vi "ProdaNG.Product.Add.vi"(8 "error in (no error)":errorcluster, 10 "Product":T1, 11 "dbHandle":i32) -> (0 "error out":errorcluster, 2 "Product out":T1, 3 "dbHandle":i32)   [LabVIEW 2016]
doc: "This function creates a new Product out of a prefilled product structure.\nParameter:\nhandle is an Integer, which is returned by the function Login() at the creation of a new connection.\nproduct is a pointer on a product structure, which elements must be prefilled. The structure must be defined and filled in the calling program. Nearly all elements of the structure must be set to reasonable values. The element id is filled by the DLL with a new Id for the created record, if the returncode is 0. The element crTime is being filled by the DLL automatically. The elements mdTime and mdProcessStepId are not being filled.\nThe function checks if a product with the passed WabcoPartId and serial number already exists and returns this. In this case no new product record is created.\nReturncodes:\n0 No error\n234 (ERROR_MORE_DATA) in case that the product already exists. This is no error and the product structure is returned with the existing product. \n< 0 ORACLE Error code\n6 (ERROR_INVALID_HANDLE) in case of an invalid handle"
uses:
  Controls/ProdaNG.Product.ctl
  Controls/ProdaNG.ProductSize.ctl
  prodllNG.dll
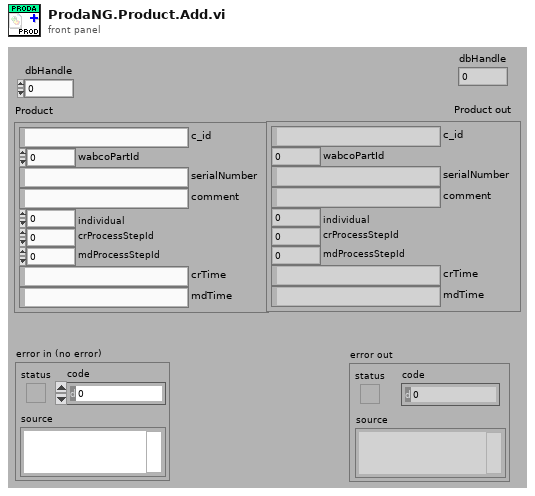
[diagram p1: front panel]
types:
  T1 = typedef "ProdaNG.Product.ctl" = cluster{"c_id":string, "wabcoPartId":i32, "serialNumber":string, "comment":string, "individual":i32, "crProcessStepId":i32, "mdProcessStepId":i32, "crTime":string, "mdTime":string}
  T2 = typedef "ProdaNG.ProductSize.ctl" = cluster{"c_id":i32, "wabcoPartId":i32, "serialNumber":i32, "comment":i32, "individual":i32, "crProcessStepId":i32, "mdProcessStepId":i32, "crTime":i32, "mdTime":i32}
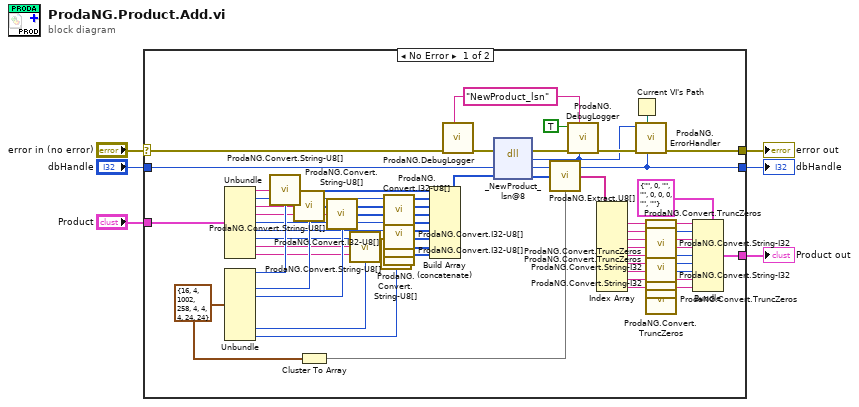
[diagram p0: block diagram]
diagram:
  n1 = case shown="No Error" "error in (no error)" {
    selector: "error in (no error)" -> [w60 w68]
    tunnel: [w66 w68] -> w5
    tunnel: "dbHandle" -> [w64 w67]
    tunnel: [w63 w67] -> w3
    tunnel: "Product" -> [w51 _]
    tunnel: [w30 _] -> w1
    frame No Error {
      w7 = T2 {"c_id"=16, "wabcoPartId"=4, "serialNumber"=1002, "comment"=258, "individual"=4, "crProcessStepId"=4, "mdProcessStepId"=4, "crTime"=24, "mdTime"=24} ("ProductSize")
      w61 = "NewProduct_lsn" ("cmd")
      n2 = Unbundle(w51) -> ("c_id"=w55:string, "wabcoPartId"=w26:i32, "serialNumber"=w25:string, "comment"=w24:string, "individual"=w18:i32, "crProcessStepId"=w16:i32, "mdProcessStepId"=w14:i32, "crTime"=w13:string, "mdTime"=w10:string)
      n3 = Unbundle(w7) -> ("c_id"=w53:i32, "serialNumber"=w23:i32, "comment"=w22:i32, "crTime"=w11:i32, "mdTime"=w9:i32)  [unwired: 4 out]
      n4 = call "ProdaNG.Convert.String-U8[].vi"("Input String"=w55, "Size"=w53) -> ("Output"=w52:u8[])
      n5 = call "ProdaNG.Convert.String-U8[].vi"("Input String"=w25, "Size"=w23) -> ("Output"=w20:u8[])
      n6 = Cluster To Array(cluster=w7) -> (array=w54:i32[])
      n7 = call "ProdaNG.Convert.String-U8[].vi"("Input String"=w24, "Size"=w22) -> ("Output"=w21:u8[])
      n8 = call "ProdaNG.Convert.String-U8[].vi"("Input String"=w13, "Size"=w11) -> ("Output"=w12:u8[])
      n9 = call "ProdaNG.Convert.String-U8[].vi"("Input String"=w10, "Size"=w9) -> ("Output"=w8:u8[])
      n10 = call "ProdaNG.Convert.I32-U8[].vi"("32bit integer"=w26) -> ("unsigned byte array"=w27:u8[])  [unwired: 10 in]
      n11 = call "ProdaNG.Convert.I32-U8[].vi"("32bit integer"=w18) -> ("unsigned byte array"=w19:u8[])  [unwired: 10 in]
      n12 = call "ProdaNG.Convert.I32-U8[].vi"("32bit integer"=w16) -> ("unsigned byte array"=w17:u8[])  [unwired: 10 in]
      n13 = call "ProdaNG.Convert.I32-U8[].vi"("32bit integer"=w14) -> ("unsigned byte array"=w15:u8[])  [unwired: 10 in]
      n14 = Build Array (concatenate)(w52, w27, w20, w21, w19, w17, w15, w12, w8) -> (w28:u8[])
      n15 = call "ProdaNG.DebugLogger.vi"("cmd"=w61, "error in (no error)"=w60) -> ("error out"=w59:errorcluster)  [unwired: 9 in]
      n16 = dll-call lib="D:/Maszup/WABCO/SVN/LineTraceSystem/SOFTWARE/sources/Database/ProdaNG/prodllNG.dll" fn="_NewProduct_lsn@8" ("ProDll.dll:InitProDll")(error in=w59, "dbHandle"=w64, "product"=w28) -> (error out=w58:errorcluster, "return type"=w56:i32, "dbHandle"=w63:i32, "product"=w29:u8[])  [unwired: 2 in, 1 out]
      n17 = call "ProdaNG.Extract.U8[].vi"("unsigned byte array"=w29, "Sizes"=w54) -> ("Elements"=w31:string[])
      n18 = call "ProdaNG.DebugLogger.vi"("return type"=w56, "cmd"=w61, "error in (no error)"=w58, "done? (F)"=TRUE) -> ("error out"=w57:errorcluster)  [unwired: 7 in]
      n19 = Index Array(array=w31) -> (element #1=w33:string, element #2=w48:string, element #3=w41:string, element #4=w40:string, element #5=w47:string, element #6=w45:string, element #7=w43:string, element #8=w37:string, element #9=w36:string)  [unwired: 9 in]
      n20 = Current VI's Path() -> (path=w65:path)
      n21 = call "ProdaNG.ErrorHandler.vi"("dbHandleIn"=w63, "Path"=w65, "error in"=w57, "output_parameter"=w56) -> ("error out"=w66:errorcluster)  [unwired: 7 in]
      n22 = call "ProdaNG.Convert.TruncZeros.vi"("string with \\0s"=w33) -> ("LV string"=w32:string)  [unwired: 10 in]
      n23 = call "ProdaNG.Convert.String-I32.vi"("unsigned byte string"=w48) -> ("32bit integer"=w49:i32)  [unwired: 10 in]
      n24 = call "ProdaNG.Convert.TruncZeros.vi"("string with \\0s"=w41) -> ("LV string"=w39:string)  [unwired: 10 in]
      n25 = call "ProdaNG.Convert.TruncZeros.vi"("string with \\0s"=w40) -> ("LV string"=w38:string)  [unwired: 10 in]
      n26 = call "ProdaNG.Convert.String-I32.vi"("unsigned byte string"=w47) -> ("32bit integer"=w46:i32)  [unwired: 10 in]
      n27 = call "ProdaNG.Convert.String-I32.vi"("unsigned byte string"=w45) -> ("32bit integer"=w44:i32)  [unwired: 10 in]
      n28 = call "ProdaNG.Convert.String-I32.vi"("unsigned byte string"=w43) -> ("32bit integer"=w42:i32)  [unwired: 10 in]
      n29 = call "ProdaNG.Convert.TruncZeros.vi"("string with \\0s"=w37) -> ("LV string"=w35:string)  [unwired: 10 in]
      n30 = call "ProdaNG.Convert.TruncZeros.vi"("string with \\0s"=w36) -> ("LV string"=w34:string)  [unwired: 10 in]
      n31 = Bundle(cluster=T1 {"c_id"="", "wabcoPartId"=0, "serialNumber"="", "comment"="", "individual"=0, "crProcessStepId"=0, "mdProcessStepId"=0, "crTime"="", "mdTime"=""} ("Product"), "c_id"=w32, "wabcoPartId"=w49, "serialNumber"=w39, "comment"=w38, "individual"=w46, "crProcessStepId"=w44, "mdProcessStepId"=w42, "crTime"=w35, "mdTime"=w34) -> (w30:T1)
    }
    frame Error {
    }
  }
  "error out" <- w5
  "dbHandle" <- w3
  "Product out" <- w1
